vi "Avg.vi"(1 "숫자형 4":i32, 2 "숫자형 3":i32, 3 "숫자형 2":i32, 4 "숫자형 1":i32) -> (0 "x/y":dbl)   [LabVIEW 2018]
doc: "4개의 숫자를 입력받아 평균을 구하는 함수"
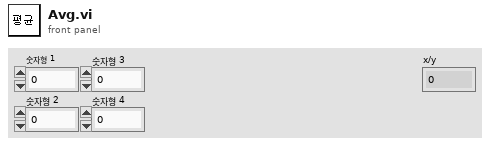
[diagram p1: front panel]
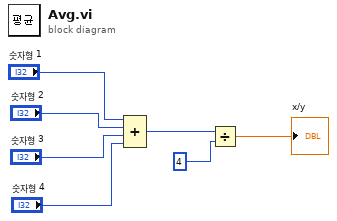
[diagram p0: block diagram]
diagram:
  n1 = Compound Arithmetic op=ADD("숫자형 1", "숫자형 2", "숫자형 3", "숫자형 4") -> (w3:i32)
  n2 = Divide(x=w3, y=4) -> (x/y=→"x/y":dbl)
